vi "GetImageSize.vi"(11 "cameraId":i32) -> (1 "Width":i32, 3 "Height":i32)   [LabVIEW 2017, in "PlayNitrideCameraComponet1010_4.lvlib"]
uses:
  <userlib>/PlayNitrideCameraComponet1010_4/PlayNitrideCameraComponet1010_4.lvlib
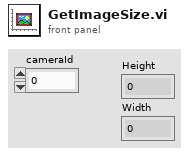
[diagram p1: front panel]
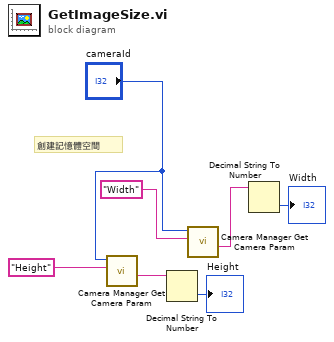
[diagram p0: block diagram]
diagram:
  # "創建記憶體空間"
  n1 = call <userlib>:"Camera Manager Get Camera Param.vi"("NodeName"="Height", "cameraId"="cameraId") -> ("Value out"=w5:string)  [unwired: 7 in, 2 out]
  n2 = Decimal String To Number(string=w5) -> (number=→"Height":i32)  [unwired: 2 in, 1 out]
  n3 = call <userlib>:"Camera Manager Get Camera Param.vi"("NodeName"="Width", "cameraId"="cameraId") -> ("Value out"=w1:string)  [unwired: 7 in, 2 out]
  n4 = Decimal String To Number(string=w1) -> (number=→"Width":i32)  [unwired: 2 in, 1 out]
